vi "吸光值计算.vi"(4 "F1":dbl, 5 "F0":dbl) -> (1 "测量吸光度":dbl)   [LabVIEW 2016, in "总磷总氮曲线模型.xctl"]
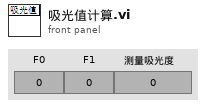
[diagram p1: front panel]
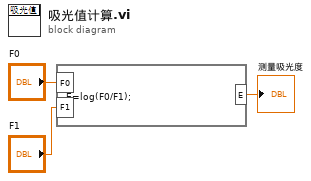
[diagram p0: block diagram]
diagram:
  n1 = formula code="E=log(F0/F1);"("F0"="F0", "F1"="F1") -> ("E"=→"测量吸光度":dbl)
